vi "Tosca-Execute Pretrial Function.vi"(0 "Pretrial in":T1, 7 "Fs":dbl, 11 "error in (no error)":errorcluster) -> (8 "output":string, 15 "error out":errorcluster)   [LabVIEW 2020]
uses:
  Typedefs/Tosca-Pretrial Spec.ctl
  Sub VIs/Tosca-Globals.vi
panel:
  out "Message":string
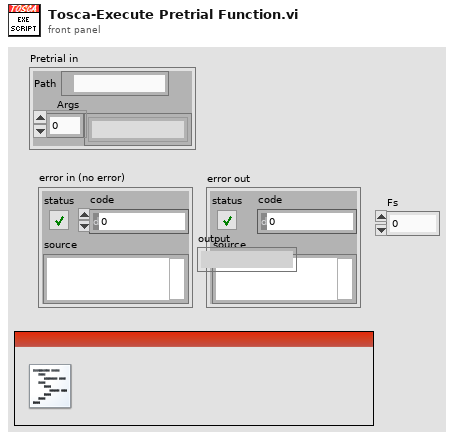
[diagram p1: front panel]
types:
  T1 = typedef "Tosca-Pretrial Spec.ctl" = cluster{"Path":path, "Args":string[]}
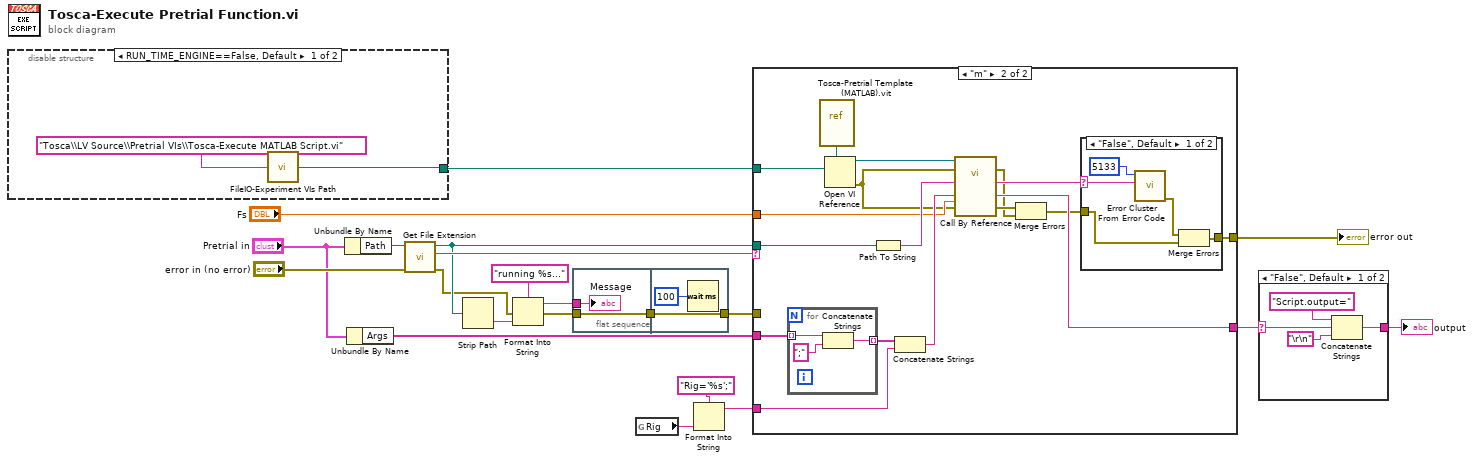
[diagram p0: block diagram]
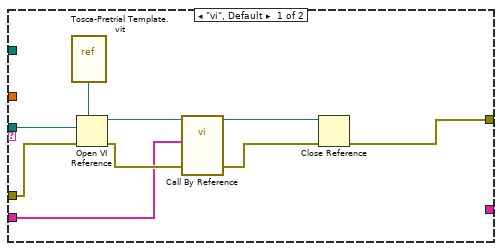
[diagram p3: hidden frame]
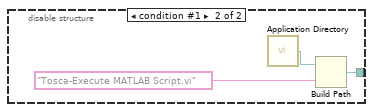
[diagram p5: hidden frame]
diagram:
  n1 = disable-structure shown="RUN_TIME_ENGINE==False, Default" {
    disable-tunnel: [w23 w24] -> w10
    frame condition #0 (active) {
      n2 = call "FileIO-Experiment VIs Path.vi"("relpath"="Tosca\\LV Source\\Pretrial VIs\\Tosca-Execute MATLAB Script.vi") -> ("full path"=w23:path)  [unwired: 4 in]
    }
    frame condition #1 {
      n3 = call <vilib>:"Application Directory.vi"() -> ("Application Directory"=w26:path)
      n4 = Build Path(base path=w26, name or relative path="Tosca-Execute MATLAB Script.vi") -> (appended path=w24:path)
    }
  }
  n5 = Unbundle By Name("Pretrial in") -> ("Path"=w21:path)
  n6 = Unbundle By Name("Pretrial in") -> ("Args"=w4:string[])
  n7 = call <vilib>:"Get File Extension.vi"("error in (no error)"="error in (no error)", "file"=w21) -> ("error out"=w9:errorcluster, "lowercase file extension"=w20:string, "dup file"=w14:path)  [unwired: 5 in, 2 out]
  n8 = Strip Path(path=w14) -> (name=w15:string)  [unwired: 1 out]
  n9 = Format Into String(format string="running %s...", error in=w9, w15) -> (resulting string=w8:string, error out=w7:errorcluster)  [unwired: 1 in]
  n10 = flat-sequence {
    tunnel: w8 -> [w28]
    tunnel: w7 -> [w27]
    tunnel: [w27] -> w6
    tunnel: w6 -> [w30]
    tunnel: [w30] -> w5
    frame #0 {
      "Message" <- w28
    }
    frame #1 {
      n11 = Wait (ms)(milliseconds to wait=u32 100) -> ()  [unwired: 1 out]
    }
  }
  n12 = global read "Tosca-Globals.vi" "Rig"() -> (w2:string)
  n13 = Format Into String(format string="Rig='%s';", w2) -> (resulting string=w1:string)  [unwired: 2 in, 1 out]
  n14 = case shown="\"m\"" w20 {
    tunnel: w5 -> [w38 _]
    tunnel: w14 -> [w39 w56]
    tunnel: [w32 w48] -> w18
    tunnel: w4 -> [w31 w55]
    tunnel: "Fs" -> [_ w51]
    tunnel: [_ w47] -> w12
    tunnel: w10 -> [_ w44]
    tunnel: w1 -> [_ w40]
    frame "vi", Default {
      n15 = vi-ref "Tosca-Pretrial Template.vit"() -> (w37:refnum<vi>)
      n16 = Open VI Reference(type specifier VI Refnum (for type only)=w37, vi path=w39, error in (no error)=w38) -> (vi reference=w36:refnum<vi>, error out=w35:errorcluster)  [unwired: 3 in]
      n17 = call-by-ref "?"(reference=w36, "Args"=w31, "error in (no error)"=w35) -> (reference out=w34:refnum<vi>, "error out"=w33:errorcluster)  [unwired: 14 in, 1 out]
      n18 = Close Reference(reference=w34, error in (no error)=w33) -> (error out=w32:errorcluster)
    }
    frame "m" {
      n19 = for {
        tunnel: w55 -> [w65] mode=indexing
        tunnel: [w63] -> w54 mode=indexing
        n20 = Concatenate Strings(w65, ";") -> (w63:string)
      }
      n21 = vi-ref "Tosca-Pretrial Template (MATLAB).vit"() -> (w41:refnum<vi>)
      n22 = Open VI Reference(type specifier VI Refnum (for type only)=w41, vi path=w44) -> (vi reference=w42:refnum<vi>, error out=w43:errorcluster)  [unwired: 4 in]
      n23 = Path To String(path=w56) -> (string=w53:string)
      n24 = Concatenate Strings(w54, w40) -> (w52:string)
      n25 = call-by-ref "?"(reference=w42, error in=w43, "Path"=w53, "Args"=w52, "Fs"=w51, 11:"error in (no error)"=w43) -> (error out=w45:errorcluster, "result"=w50:string, "output"=w47:string, 15:"error out"=w49:errorcluster)  [unwired: 9 in, 1 out]
      n26 = Merge Errors(w49, w45) -> (w46:errorcluster)
      n27 = case shown="\"False\", Default" w50 {
        selector: w50 -> [w59 _]
        tunnel: w46 -> [w60 w62]
        tunnel: [w61 w62] -> w48
        frame "False", Default {
          n28 = call <vilib>:"Error Cluster From Error Code.vi"("error message (\"\")"=w59, "error code (0)"=5133) -> ("error out"=w58:errorcluster)  [unwired: 7 in]
          n29 = Merge Errors(w58, w60) -> (w61:errorcluster)
        }
        frame "" {
        }
      }
    }
  }
  "error out" <- w18
  n30 = case shown="\"False\", Default" w12 {
    selector: w12 -> [w69 w70]
    tunnel: [w68 w70] -> w11
    frame "False", Default {
      n31 = Concatenate Strings("Script.output=" ("string"), w69, "\r\n") -> (w68:string)
    }
    frame "" {
    }
  }
  "output" <- w11
